vi "Lab4.vi"() -> ()   [LabVIEW 2021]
panel:
  in  "stop":bool
  out "Number":dbl
  out "Green":bool
  out "Yellow":bool
  out "Red":bool
  # "Traffic Light"
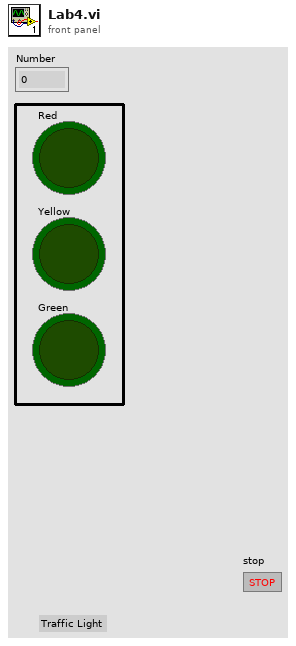
[diagram p1: front panel]
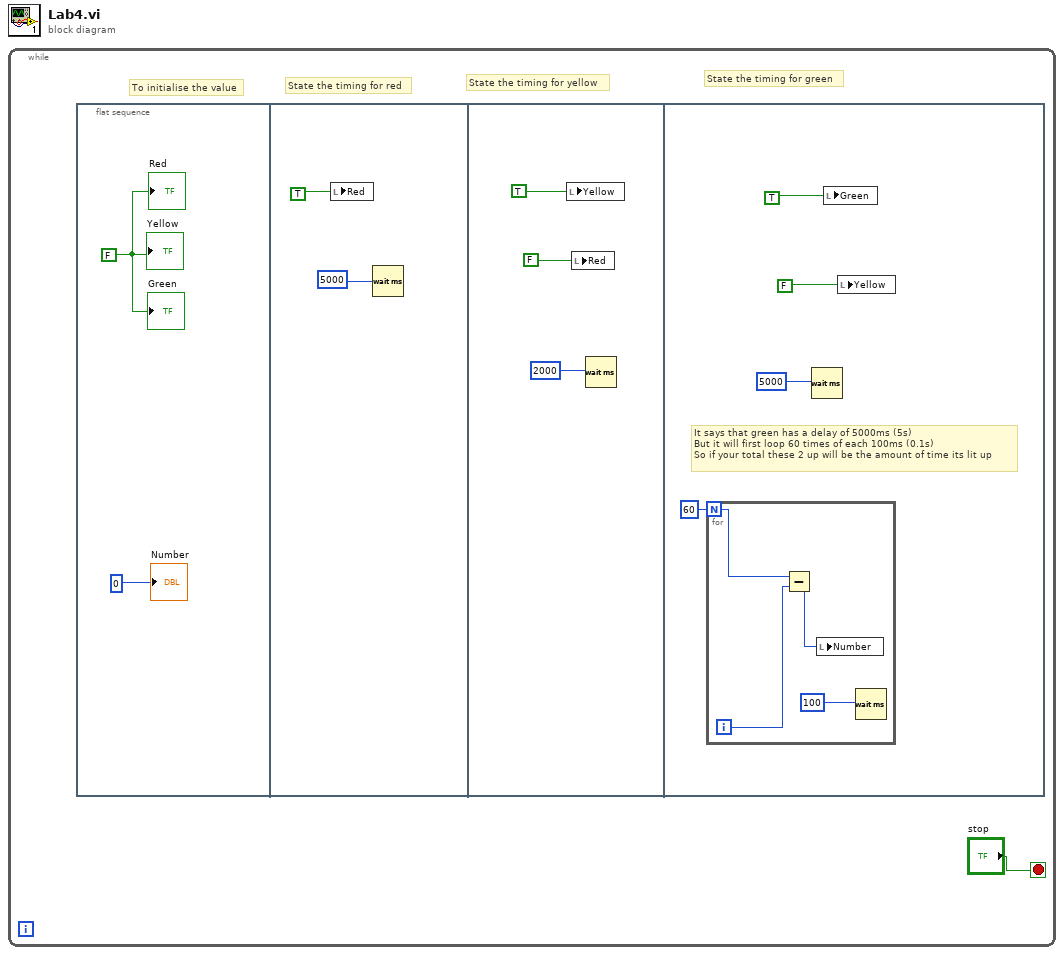
[diagram p0: block diagram]
diagram:
  n1 = while {
    stop <- "stop" stop-if-true
    # "State the timing for green"
    # "State the timing for yellow"
    # "State the timing for red"
    # "To initialise the value"
    n2 = flat-sequence {
      frame #0 {
        w2 = FALSE
        "Number" <- 0
        "Red" <- w2
        "Yellow" <- w2
        "Green" <- w2
      }
      frame #1 {
        n3 = local write "Red"(TRUE) -> ()
        n4 = Wait (ms)(milliseconds to wait=5000) -> ()  [unwired: 1 out]
      }
      frame #2 {
        n5 = local write "Yellow"(TRUE) -> ()
        n6 = local write "Red"(FALSE) -> ()
        n7 = Wait (ms)(milliseconds to wait=2000) -> ()  [unwired: 1 out]
      }
      frame #3 {
        # "It says that green has a delay of 5000ms (5s)\nBut it will first loop 60 times of each 100ms (0.1s)\nSo if your total these 2 up will be the amount of time its lit up"
        n8 = for {
          N: 60 -> [w16]
          i -> [w15]
          n9 = Subtract(x=w16, y=w15) -> (x-y=w14:i32)
          n10 = local write "Number"(w14) -> ()
          n11 = Wait (ms)(milliseconds to wait=100) -> ()  [unwired: 1 out]
        }
        n12 = Wait (ms)(milliseconds to wait=5000) -> ()  [unwired: 1 out]
        n13 = local write "Green"(TRUE) -> ()
        n14 = local write "Yellow"(FALSE) -> ()
      }
    }
  }
